vi "vending machine.vi"() -> ()   [LabVIEW 2015]
uses:
  numeric display.ctl
  Control 4.ctl
panel:
  out "vend?":bool
  in  "20":dbl
  in  "21":dbl
  in  "10":dbl
  in  "11":dbl
  out "sevensegdisplay":T1 format="%_3g"
  out "No. of coins returned":i32[](array[numeric])
  out "action":string
  in  "Controls 2":T2
  in  "Controls 3":T3
  # "price stored in pence"
  # "machine vends coins \nin order shown in array.\n1 pound\n50p\n20p\n10p\n5p"
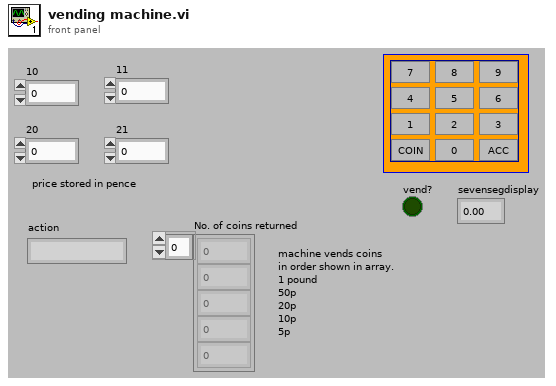
[diagram p1: front panel]
types:
  T1 = typedef "numeric display.ctl" = dbl
  T2 = cluster{"0":bool, "1":bool, "2":bool, "3":bool, "4":bool, "5":bool, "6":bool, "7":bool, "8":bool, "9":bool, "ACCEPT":bool, "CHANGE":bool, "Action":bool}
  T3 = cluster{"Up":bool, "Left":bool, "Down":bool, "Right":bool, "Action":bool}
  T4 = typedef "Control 4.ctl" = cluster{"Up":refnum<vi>, "Left":refnum<vi>, "Down":refnum<vi>, "Right":refnum<vi>, "Right 2":refnum<vi>, "Down 2":refnum<vi>, "Left 2":refnum<vi>, "Up 2":refnum<vi>, "Right 3":refnum<vi>, "Down 3":refnum<vi>, "Left 3":refnum<vi>, "Up 3":refnum<vi>}
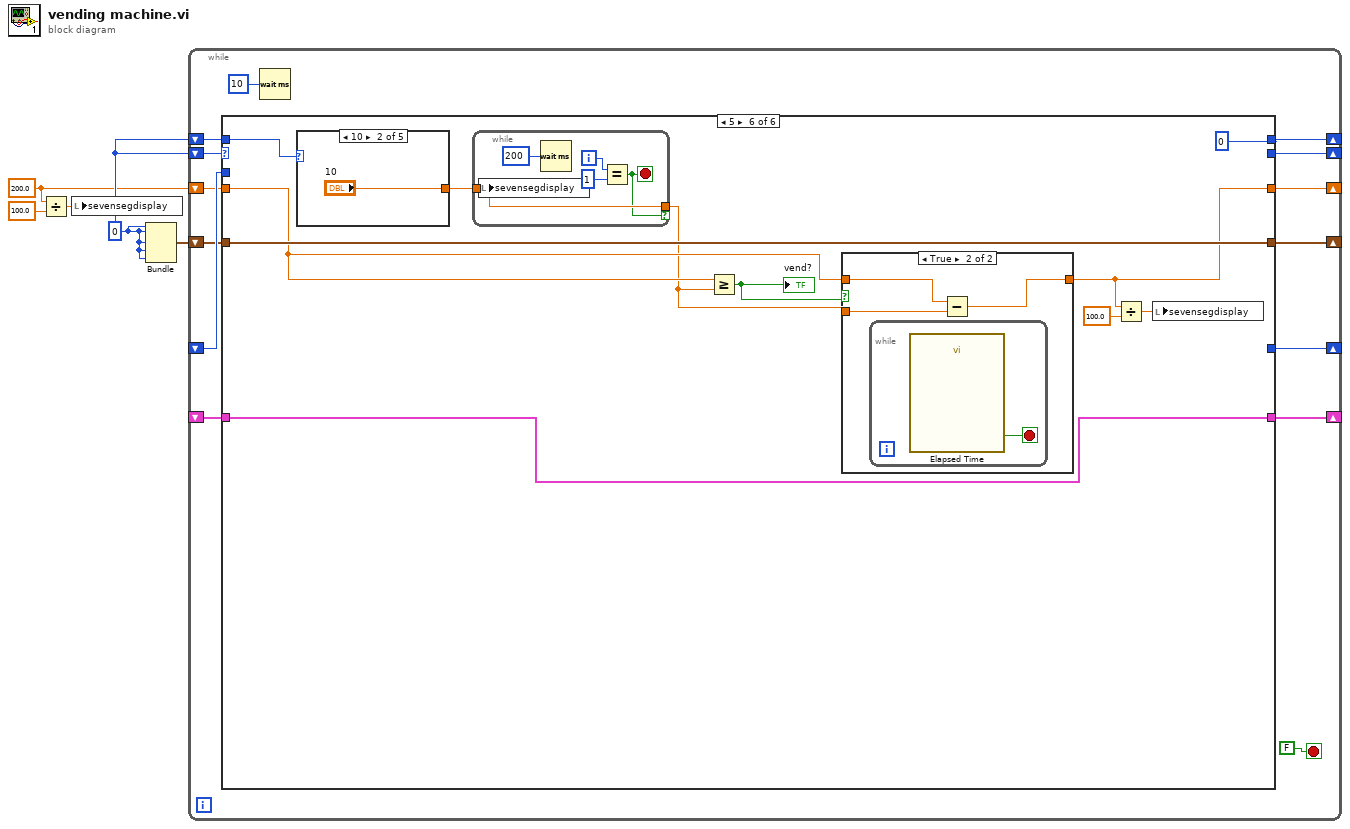
[diagram p0: block diagram]
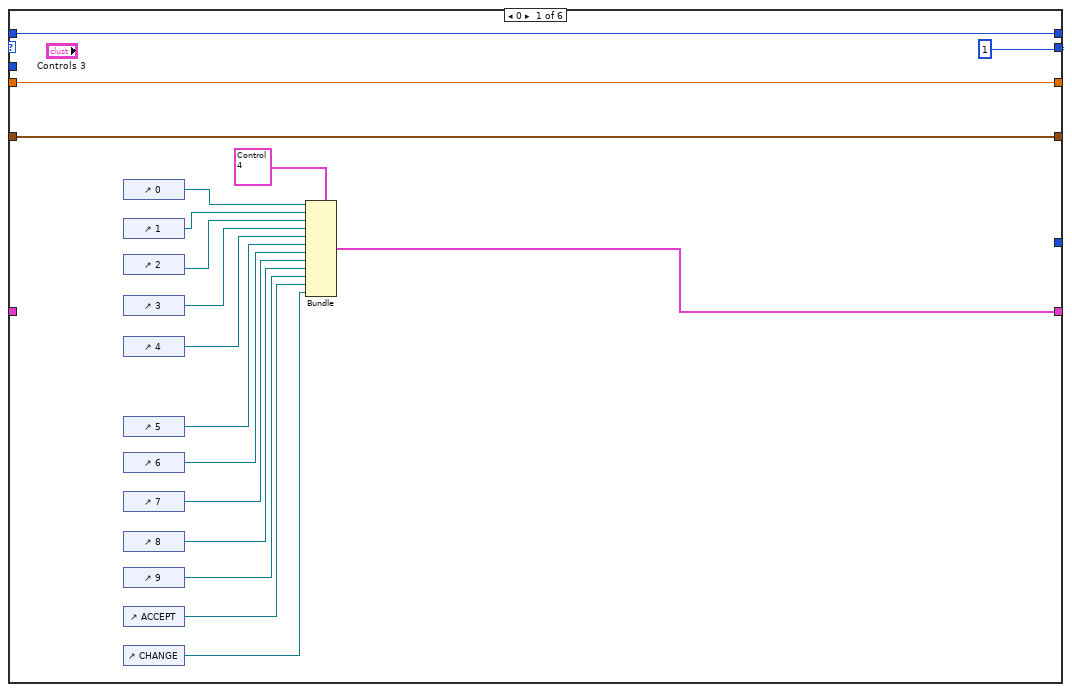
[diagram p2: hidden frame]
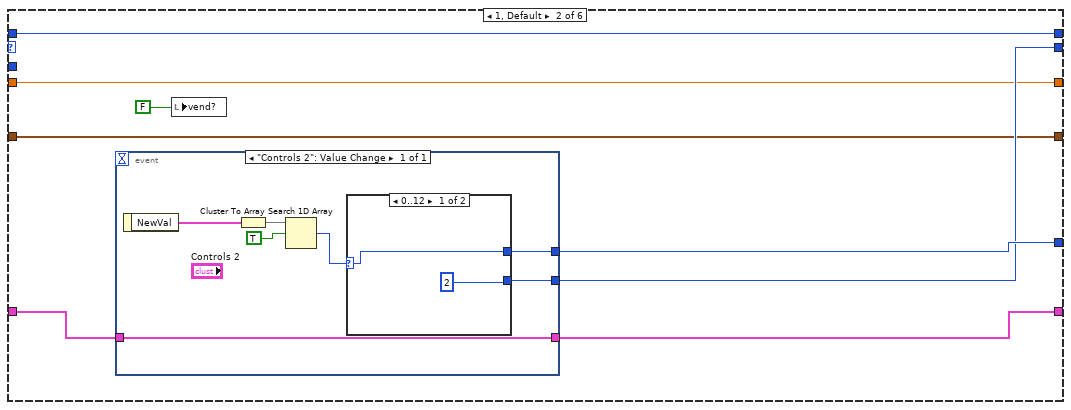
[diagram p3: hidden frame]
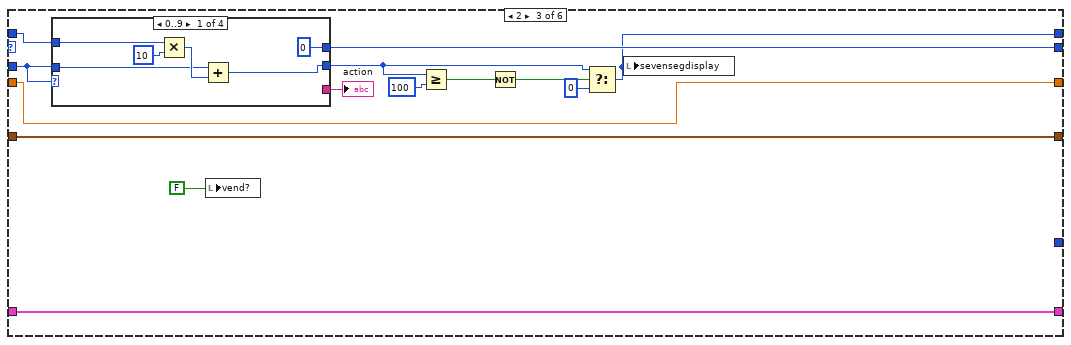
[diagram p5: hidden frame]
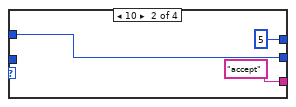
[diagram p6: hidden frame]
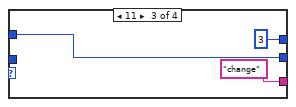
[diagram p7: hidden frame]
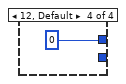
[diagram p8: hidden frame]
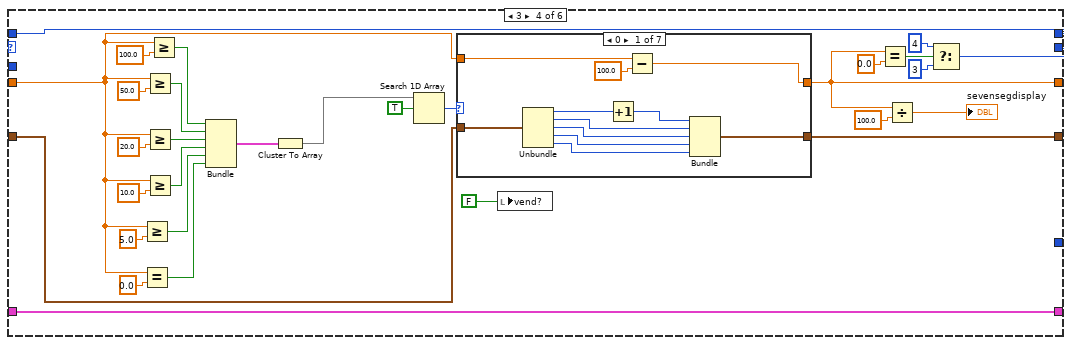
[diagram p9: hidden frame]
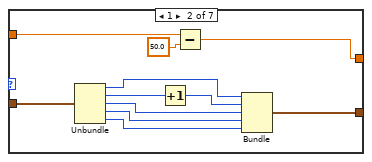
[diagram p10: hidden frame]
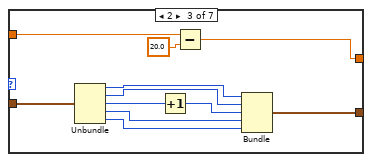
[diagram p11: hidden frame]
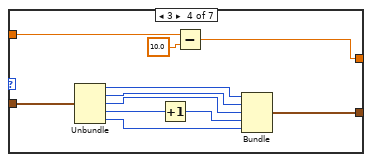
[diagram p12: hidden frame]
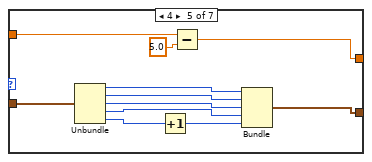
[diagram p13: hidden frame]
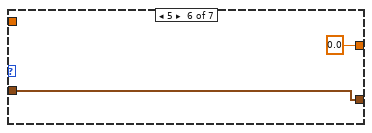
[diagram p14: hidden frame]
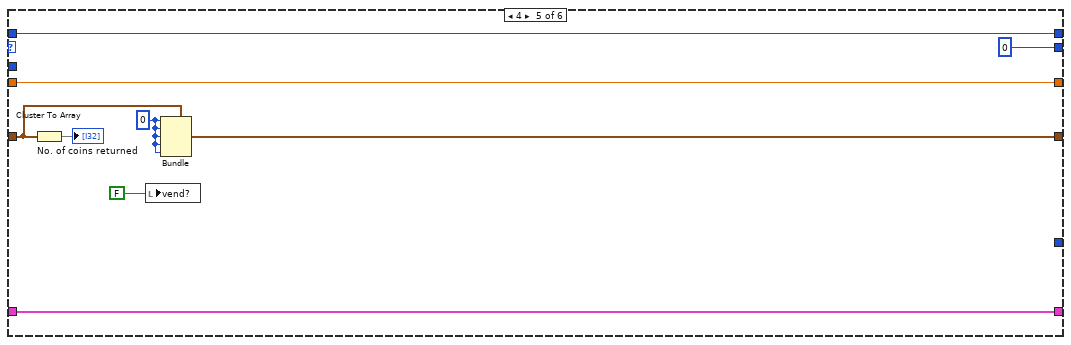
[diagram p16: hidden frame]
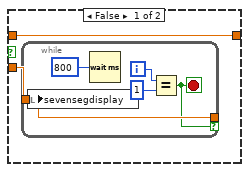
[diagram p17: hidden frame]
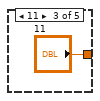
[diagram p19: hidden frame]
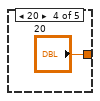
[diagram p20: hidden frame]
diagram:
  w4 = 0
  w1 = 200.0
  n1 = Divide(x=w1, y=100.0) -> (x/y=w3:dbl)
  n2 = local write "sevensegdisplay"(w3) -> ()
  n3 = Bundle(w4, w4, w4, w4, w4) -> (w5:cluster{i32, i32, i32, i32, i32})  [unwired: 1 in]
  n4 = while {
    shift-right: [w12] -> _
    shift-left: w4 -> [w15]
    shift-right: [w13] -> _
    shift-left: _ -> [w14]
    shift-right: [w18] -> _
    shift-left: _ -> [w19]
    shift-right: [w11] -> _
    shift-left: w4 -> [w10]
    shift-right: [w6] -> _
    shift-left: w1 -> [w9]
    shift-right: [w7] -> _
    shift-left: w5 -> [w8]
    stop <- FALSE stop-if-true
    n5 = case shown="5" w15 {
      tunnel: [1 w42 w57 w95 0 _] -> w12
      tunnel: [_ w43 _ _ _ _] -> w13
      tunnel: w19 -> [_ w45 w68 w101 w178 w190]
      tunnel: [w36 w44 w68 w101 w178 w190] -> w18
      tunnel: w14 -> [_ _ w65 _ _ _]
      tunnel: [w22 w41 w56 w83 w172 0] -> w11
      tunnel: w10 -> [w22 w41 w64 w83 w172 w188]
      tunnel: [w20 w40 w67 w92 w179 w181] -> w6
      tunnel: w9 -> [w20 w40 w67 w88 w179 w186]
      tunnel: w8 -> [w21 w39 w66 w98 w175 w189]
      tunnel: [w21 w39 w66 w97 w177 w189] -> w7
      frame 0 {
        n6 = control-ref of="0"() -> (w34:refnum<vi>)
        n7 = control-ref of="1"() -> (w33:refnum<vi>)
        n8 = control-ref of="2"() -> (w32:refnum<vi>)
        n9 = control-ref of="3"() -> (w31:refnum<vi>)
        n10 = control-ref of="4"() -> (w30:refnum<vi>)
        n11 = control-ref of="5"() -> (w29:refnum<vi>)
        n12 = control-ref of="6"() -> (w28:refnum<vi>)
        n13 = control-ref of="7"() -> (w27:refnum<vi>)
        n14 = control-ref of="8"() -> (w26:refnum<vi>)
        n15 = control-ref of="9"() -> (w25:refnum<vi>)
        n16 = control-ref of="ACCEPT"() -> (w24:refnum<vi>)
        n17 = control-ref of="CHANGE"() -> (w23:refnum<vi>)
        n18 = Bundle(cluster=T4 {"Up"=refnum, "Left"=refnum, "Down"=refnum, "Right"=refnum, "Right 2"=refnum, "Down 2"=refnum, "Left 2"=refnum, "Up 2"=refnum, "Right 3"=refnum, "Down 3"=refnum, "Left 3"=refnum, "Up 3"=refnum}, "Up"=w34, "Left"=w33, "Down"=w32, "Right"=w31, "Right 2"=w30, "Down 2"=w29, "Left 2"=w28, "Up 2"=w27, "Right 3"=w26, "Down 3"=w25, "Left 3"=w24, "Up 3"=w23) -> (w36:T4)
      }
      frame 1, Default {
        n19 = event shown="[0] \"Controls 2\": Value Change" {
          selector: _ -> [_]
          dyn-events: _ -> [_]
          timeout: _ -> [_]
          tunnel: [w52] -> w42
          tunnel: [w46] -> w44
          tunnel: [w47] -> w43
          tunnel: w45 -> [w46]
          event "Controls 2": Value Change {
            n20 = event-data() -> ("NewVal"=w48:T2)  [unwired: 1 in]
            n21 = Cluster To Array(cluster=w48) -> (array=w51:bool[])
            n22 = Search 1D Array(1D array=w51, element=TRUE) -> (index of element=w49:i32)  [unwired: 1 in]
            n23 = case shown="0..12" w49 {
              selector: w49 -> [w53 _]
              tunnel: [2 _] -> w52
              tunnel: [w53 _] -> w47
              frame 0..12 {
                # "Direction pressed"
              }
              frame Default {
                # "This shouldn't happen"
              }
            }
          }
        }
        n24 = local write "vend?"(FALSE ("vend? 2")) -> ()
      }
      frame 2 {
        n25 = case shown="0..9" w65 {
          tunnel: [w69 w75 w78 _] -> w59
          tunnel: [_ "accept" "change" _] -> w58
          tunnel: [0 5 3 0] -> w57
          tunnel: w65 -> [w70 _ _ _]
          tunnel: w64 -> [w72 w75 w78 _]
          frame 0..9 {
            n26 = Multiply(x=w72, y=10) -> (x*y=w71:i32)
            n27 = Add(x=w70, y=w71) -> (x+y=w69:i32)
          }
          frame 10 {
          }
          frame 11 {
          }
          frame 12, Default {
          }
        }
        "action" <- w58
        n28 = local write "vend?"(FALSE ("vend? 2")) -> ()
        n29 = Greater Or Equal?(x=w59, y=100) -> (x >= y?=w61:bool)
        n30 = Not(x=w61) -> (.not. x?=w63:bool)
        n31 = Select(t=w59, s=w63, f=0) -> (s? t:f=w56:i32)
        n32 = local write "sevensegdisplay"(w56) -> ()
      }
      frame 3 {
        n33 = Greater Or Equal?(x=w88, y=5.0) -> (x >= y?=w86:bool)
        n34 = Equal?(x=w88, y=0.0) -> (x = y?=w90:bool)
        n35 = Greater Or Equal?(x=w88, y=50.0) -> (x >= y?=w106:bool)
        n36 = Greater Or Equal?(x=w88, y=20.0) -> (x >= y?=w105:bool)
        n37 = Greater Or Equal?(x=w88, y=10.0) -> (x >= y?=w104:bool)
        n38 = Greater Or Equal?(x=w88, y=100.0) -> (x >= y?=w107:bool)
        n39 = Bundle(w107, w106, w105, w104, w86, w90) -> (w87:cluster{bool, bool, bool, bool, bool, bool})  [unwired: 1 in]
        n40 = Cluster To Array(cluster=w87) -> (array=w103:bool[])
        n41 = Search 1D Array(1D array=w103, element=TRUE) -> (index of element=w99:i32)  [unwired: 1 in]
        n42 = case shown="0" w99 {
          tunnel: w88 -> [w122 w132 w143 w154 w165 _ w170]
          tunnel: [w120 w131 w142 w153 w164 0.0 ("y") w170] -> w92
          tunnel: w98 -> [w114 w125 w136 w152 w158 w168 w169]
          tunnel: [w113 w124 w135 w146 w157 w168 w169] -> w97
          frame 0 {
            n43 = Unbundle(w114) -> (w119:i32, w118:i32, w117:i32, w116:i32, w115:i32)
            n44 = Increment(x=w119) -> (x+1=w112:i32)
            n45 = Subtract(x=w122, y=100.0) -> (x-y=w120:dbl)
            n46 = Bundle(w112, w118, w117, w116, w115) -> (w113:cluster{i32, i32, i32, i32, i32})  [unwired: 1 in]
          }
          frame 1 {
            n47 = Unbundle(w125) -> (w130:i32, w129:i32, w128:i32, w127:i32, w126:i32)
            n48 = Increment(x=w129) -> (x+1=w123:i32)
            n49 = Subtract(x=w132, y=50.0) -> (x-y=w131:dbl)
            n50 = Bundle(w130, w123, w128, w127, w126) -> (w124:cluster{i32, i32, i32, i32, i32})  [unwired: 1 in]
          }
          frame 2 {
            n51 = Unbundle(w136) -> (w141:i32, w140:i32, w139:i32, w138:i32, w137:i32)
            n52 = Increment(x=w139) -> (x+1=w134:i32)
            n53 = Subtract(x=w143, y=20.0) -> (x-y=w142:dbl)
            n54 = Bundle(w141, w140, w134, w138, w137) -> (w135:cluster{i32, i32, i32, i32, i32})  [unwired: 1 in]
          }
          frame 3 {
            n55 = Unbundle(w152) -> (w151:i32, w150:i32, w149:i32, w148:i32, w147:i32)
            n56 = Increment(x=w148) -> (x+1=w145:i32)
            n57 = Subtract(x=w154, y=10.0) -> (x-y=w153:dbl)
            n58 = Bundle(w151, w150, w149, w145, w147) -> (w146:cluster{i32, i32, i32, i32, i32})  [unwired: 1 in]
          }
          frame 4 {
            n59 = Unbundle(w158) -> (w163:i32, w162:i32, w161:i32, w160:i32, w159:i32)
            n60 = Increment(x=w159) -> (x+1=w156:i32)
            n61 = Subtract(x=w165, y=5.0) -> (x-y=w164:dbl)
            n62 = Bundle(w163, w162, w161, w160, w156) -> (w157:cluster{i32, i32, i32, i32, i32})  [unwired: 1 in]
          }
          frame 5 {
          }
          frame 6, Default {
          }
        }
        n63 = local write "vend?"(FALSE ("vend? 2")) -> ()
        n64 = Equal?(x=w92, y=0.0) -> (x = y?=w94:bool)
        n65 = Divide(x=w92, y=100.0) -> (x/y=→"sevensegdisplay":dbl)
        n66 = Select(t=4, s=w94, f=3 ("index of element")) -> (s? t:f=w95:i32)
      }
      frame 4 {
        w176 = 0
        n67 = Cluster To Array(cluster=w175) -> (array=→"No. of coins returned":i32[])
        n68 = local write "vend?"(FALSE ("vend? 2")) -> ()
        n69 = Bundle(cluster=w175, w176, w176, w176, w176, w176) -> (w177:cluster{i32, i32, i32, i32, i32})
      }
      frame 5 {
        n70 = case shown="10" w188 {
          tunnel: [_ "10" "11" "20" "21"] -> w185
          frame 0, Default {
          }
          frame 10 {
          }
          frame 11 {
          }
          frame 20 {
          }
          frame 21 {
          }
        }
        n71 = while {
          tunnel: w185 -> [w203]
          tunnel: [w203] -> w180 if=w202
          i -> [w205]
          stop <- w202 stop-if-true
          n72 = local write "sevensegdisplay"(w203) -> ()
          n73 = Wait (ms)(milliseconds to wait=u32 200) -> ()  [unwired: 1 out]
          n74 = Equal?(x=w205, y=1) -> (x = y?=w202:bool)
        }
        n75 = Greater Or Equal?(x=w186, y=w180) -> (x >= y?=w184:bool)
        "vend?" <- w184
        n76 = case shown="True" w184 {
          tunnel: [w192 w198] -> w181
          tunnel: w186 -> [w192 w199]
          tunnel: w180 -> [w191 w200]
          frame False {
            n77 = while {
              tunnel: w191 -> [w194]
              tunnel: [w194] -> _ if=w193
              i -> [w196]
              stop <- w193 stop-if-true
              n78 = local write "sevensegdisplay"(w194) -> ()
              n79 = Wait (ms)(milliseconds to wait=u32 800) -> ()  [unwired: 1 out]
              n80 = Equal?(x=w196, y=1) -> (x = y?=w193:bool)
            }
          }
          frame True {
            n81 = while {
              stop <- w201 stop-if-true
              n82 = call "Elapsed Time"() -> ("Time has Elapsed"=w201:bool)  [unwired: 12 in, 7 out]
            }
            n83 = Subtract(x=w199, y=w200) -> (x-y=w198:dbl)
          }
        }
        n84 = Divide(x=w181, y=100.0) -> (x/y=w183:dbl)
        n85 = local write "sevensegdisplay"(w183) -> ()
      }
    }
    n86 = Wait (ms)(milliseconds to wait=u32 10) -> ()  [unwired: 1 out]
  }
